vi "Start Continuous Test Cycles [STP].vi"(7 "Micropulse # In":i32, 8 "error in (no error)":errorcluster, 11 "Test Number":u32 caption="Test Number (def: 0, all tests)") -> (0 "error out":errorcluster, 5 "Micropulse # Out":i32)   [LabVIEW 2026, in "MicroPulse_Driver.lvlib"]
doc: "The specified test(s) is repeated until a new mode (for example: STL or STX) is requested. The data is buffered for each cycle, i.e. if a single test is requested then data is output between each test, if all tests requested then data for each cycle of tests is buffered and output. The tests within a cycle are fired at the requested PRF (subject to gates set not being longer than the PRF). The next cycle will not start until this data has been output.\nParameters:\n<Tn> : Test number. An integer value from 0 to the maximum number of tests (default maximum is 1279 tests).\nTn = 0 for all conventional tests. If the S extension is used it applies to all tests in the sweep number specified: 1-32, 0 = all sweeps\n\nExample:\nNUM 100\nSTP 0 : MicroPulse sends data for tests 1 to 100 repeatedly\nSTL 1 : After completing the reporting of the data from the last test cycle, the MicroPulse enters STL mode on test 1."
uses:
  MicroPulse_Driver.lvlib
  Private/MP-Registry Action-Enum.ctl
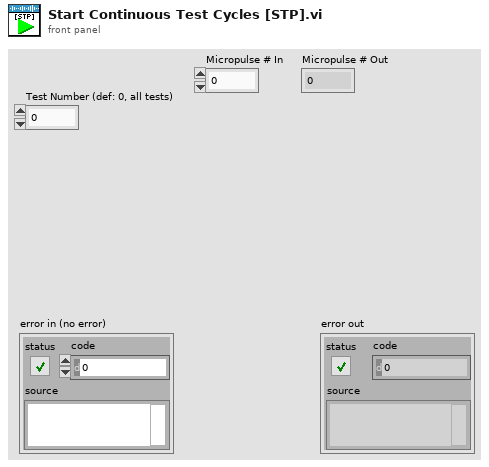
[diagram p1: front panel]
types:
  T1 = typedef "MicroPulse_Driver.lvlib/TCP config.ctl" = cluster{"Connection ID":refnum<k5>, "IP address":string, "host port":u16, "OC timeout":i32, "Read timeout":i32, "Write timeout":i32}
  T2 = typedef "MicroPulse_Driver.lvlib/MP-Registry Action-Enum.ctl" = enum16{"Read", "Add Test", "Add Command", "Add Gate Command", "Add Encoder Command", "Clear Command  List", "Set Registry", "Set System Details", "Set DOF", "Set Velocity", "Disable Asynch Reads", "Enable Asynch Reads", "Add Connection", "Disconnect", "Shutdown"}
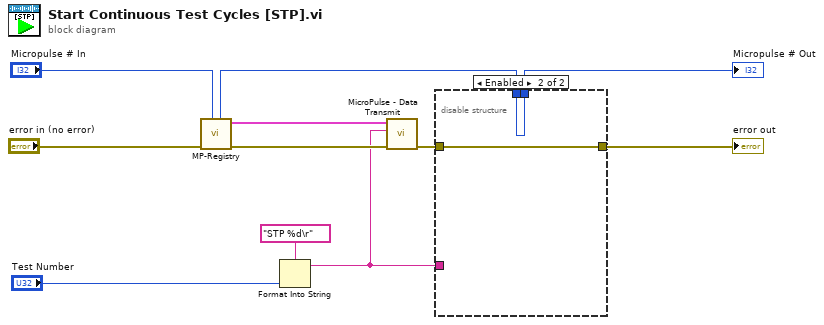
[diagram p0: block diagram]
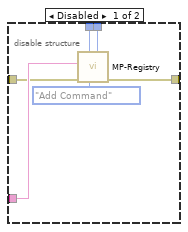
[diagram p2: hidden frame]
diagram:
  n1 = call "MP-Registry.vi"("Micropulse # In"="Micropulse # In", "error in (no error)"="error in (no error)") -> ("error out"=w9:errorcluster, "TCP config"=w8:T1, "Micropulse # Out"=w3:i32)  [unwired: 6 in, 1 out]
  n2 = Format Into String(format string="STP %d\r", "Test Number") -> (resulting string=w6:string)  [unwired: 2 in, 1 out]
  n3 = call "MicroPulse - Data Transmit.vi"("error in (no error)"=w9, "data"=w6, "TCP config"=w8) -> ("error out"=w5:errorcluster)  [unwired: 6 in, 2 out]
  n4 = disable-structure shown="Enabled" {
    disable-tunnel: w6 -> [w17 _]
    disable-tunnel: w5 -> [w15 w18]
    disable-tunnel: [w14 w18] -> w4
    disable-tunnel: w3 -> [w13 w19]
    disable-tunnel: [w12 w19] -> w2
    frame Disabled {
      n5 = call "MP-Registry.vi"("Action"=MP-Registry_Action-Enum."Add Command", "Micropulse # In"=w13, "error in (no error)"=w15, "Data in"=w17) -> ("error out"=w14:errorcluster, "Micropulse # Out"=w12:i32)  [unwired: 4 in, 2 out]
    }
    frame Enabled {
    }
  }
  "error out" <- w4
  "Micropulse # Out" <- w2
